vi "Performance Test.vi"() -> ()   [LabVIEW 2013]
uses:
  src/JKI JSON Serialization.lvlib
panel:
  out "LV Unflatten":u32(graph)
  out "LV Unflatten":u32
  out "Unflatten":u32(graph)
  out "Flatten":u32(graph)
  out "Unflatten":u32
  out "Flatten":u32
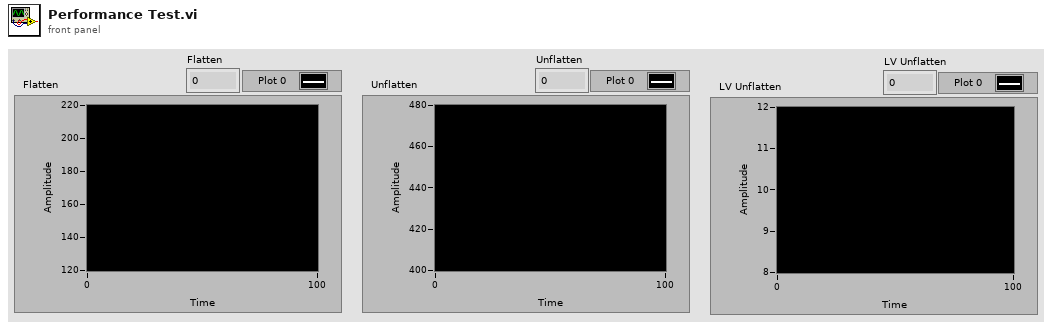
[diagram p1: front panel]
types:
  T1 = cluster{"Name":string, "Value":i32, "Array":dbl[]}[]
  T2 = cluster{"Name":string, "Value":i32, "Array":dbl[]}
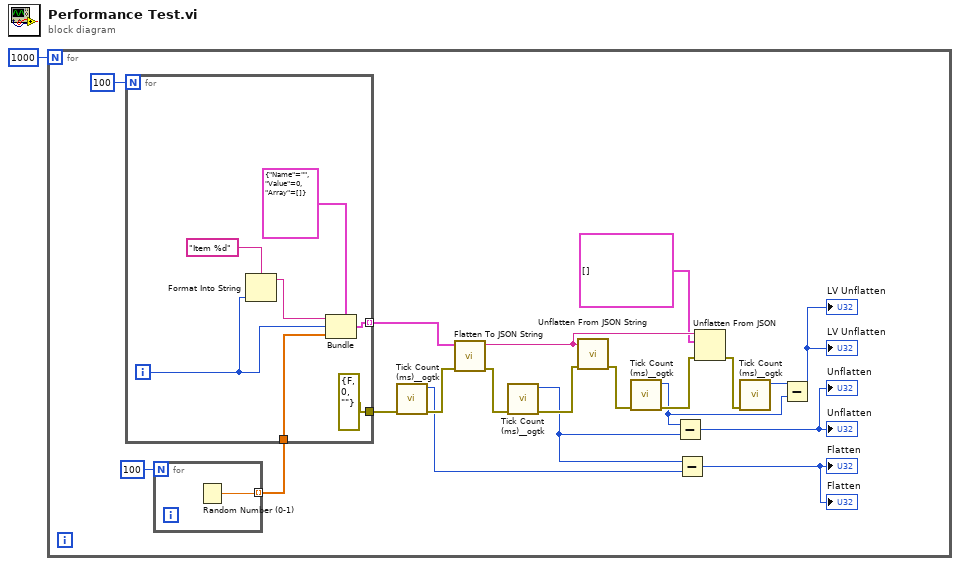
[diagram p0: block diagram]
diagram:
  n1 = for {
    N: 1000 -> [_]
    n2 = for {
      N: 100 -> [_]
      tunnel: [w22] -> w4 mode=indexing
      n3 = Random Number (0-1)() -> (number: 0 to 1=w22:dbl)
    }
    n4 = for {
      N: 100 -> [_]
      tunnel: [w25] -> w6 mode=indexing
      tunnel: [errorcluster {"status"=FALSE, "code"=0, "source"=""} ("error in (no error)")] -> w18
      tunnel: w4 -> [w23]
      i -> [w27]
      n5 = Format Into String(format string="Item %d", w27) -> (resulting string=w28:string)  [unwired: 2 in, 1 out]
      n6 = Bundle(cluster=T2 {"Name"="", "Value"=0, "Array"=[]}, "Name"=w28, "Value"=w27, "Array"=w23) -> (w25:T2)
    }
    n7 = call <userlib>:"Tick Count (ms)__ogtk.vi"("error in (no error)"=w18) -> ("error out"=w21:errorcluster, "millisecond timer value"=w15:u32)  [unwired: 9 in]
    n8 = call "Flatten To JSON String.vi"("error in (no error)"=w21, "Variant"=w6) -> ("error out"=w20:errorcluster, "JSON String"=w5:string)  [unwired: 8 in]
    n9 = call <userlib>:"Tick Count (ms)__ogtk.vi"("error in (no error)"=w20) -> ("error out"=w19:errorcluster, "millisecond timer value"=w16:u32)  [unwired: 9 in]
    n10 = call "Unflatten From JSON String.vi"("error in (no error)"=w19, "JSON String"=w5) -> ("error out"=w17:errorcluster)  [unwired: 8 in, 1 out]
    n11 = call <userlib>:"Tick Count (ms)__ogtk.vi"("error in (no error)"=w17) -> ("error out"=w13:errorcluster, "millisecond timer value"=w10:u32)  [unwired: 9 in]
    n12 = Subtract(x=w10, y=w16) -> (x-y=→"Unflatten" →"Unflatten":u32)
    n13 = Subtract(x=w16, y=w15) -> (x-y=→"Flatten" →"Flatten":u32)
    n14 = Unflatten From JSON(JSON string=w5, type and defaults=T1 [], error in (no error)=w13) -> (error out=w12:errorcluster)  [unwired: 4 in, 1 out]
    n15 = call <userlib>:"Tick Count (ms)__ogtk.vi"("error in (no error)"=w12) -> ("millisecond timer value"=w11:u32)  [unwired: 9 in, 1 out]
    n16 = Subtract(x=w11, y=w10) -> (x-y=→"LV Unflatten" →"LV Unflatten":u32)
  }
